vi "Initialize_Control_JL.vi"(0 "ERD Loop":refnum<queue>, 2 "GEA2":refnum<queue>, 5 "Receive Loop":refnum<user-event>, 7 "UI Loop Error":refnum<user-event>, 11 "Error In":errorcluster) -> (15 "Error Out":errorcluster)   [LabVIEW 2023]
uses:
  Common/type defs/ERD_Data_Loop_Control.ctl
  Common/type defs/ERD_Loop_States.ctl
  Common/GExplorer Support/typedefs/GExplorer_Data_Cluster.ctl
  Common/type defs/Error_Command.ctl
  Common/type defs/ERD_Loop_Control_Command.ctl
  Common/type defs/GEA2_Control_Command.ctl
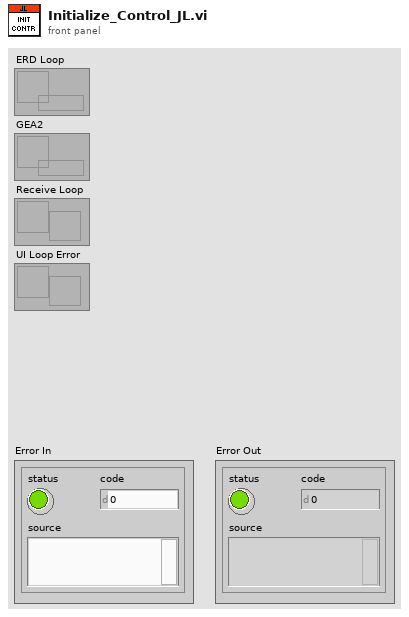
[diagram p1: front panel]
types:
  T1 = typedef "GEA2_Control_Command.ctl" = enum16{"Initialize", "Shutdown"}
  T2 = typedef "ERD_Loop_Control_Command.ctl" = enum16{"Initialize", "Shutdown"}
  T3 = typedef "Error_Command.ctl" = enum16{"Initialize", "Handle Errors", "Report Errors"}
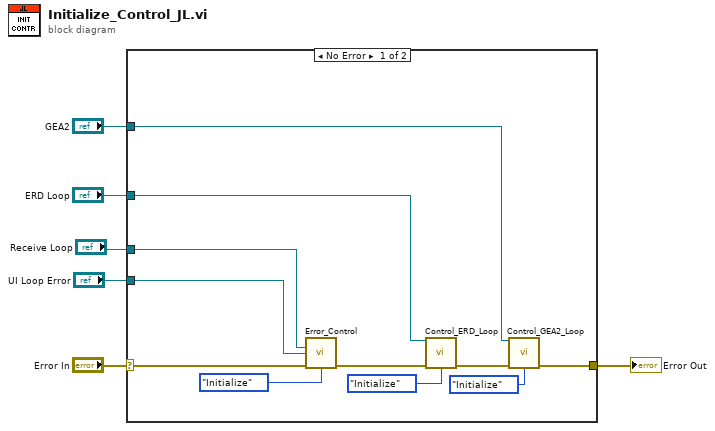
[diagram p0: block diagram]
diagram:
  n1 = case shown="No Error" "Error In" {
    selector: "Error In" -> [w12 w18]
    tunnel: [w7 w18] -> w5
    tunnel: "Receive Loop" -> [w8 _]
    tunnel: "ERD Loop" -> [w11 _]
    tunnel: "GEA2" -> [w10 _]
    tunnel: "UI Loop Error" -> [w9 _]
    frame No Error {
      n2 = call "Error_Control.vi"("Command (Handle Errors)"=Error_Command."Initialize", "Receive Loop"=w8, "UI Loop Error"=w9, "Error In"=w12) -> ("Error Out"=w13:errorcluster)  [unwired: 11 in]
      n3 = call "Control_ERD_Loop.vi"("ERD Loop"=w11, "Command (ERD Loop Control)"=ERD_Loop_Control_Command."Initialize", "Error In"=w13) -> ("Error Out"=w15:errorcluster)  [unwired: 12 in]
      n4 = call "Control_GEA2_Loop.vi"("GEA2"=w10, "Command (ERD Loop Control)"=GEA2_Control_Command."Initialize", "Error In"=w15) -> ("Error Out"=w7:errorcluster)  [unwired: 12 in]
    }
    frame Error {
    }
  }
  "Error Out" <- w5
